vi "Frame Description FGV [Body Index].vi"(8 "error in (no error)":errorcluster, 9 "Command":enum16{"Get", "Set"}(ring)=enum."Set", 10 "FrameDescription":T1) -> (0 "error out":errorcluster, 2 "FrameDescription":T1)   [LabVIEW 2011, in "KinectOne.lvlib"]
uses:
  KinectOne.lvlib
  Type Defs/FrameDescription.ctl
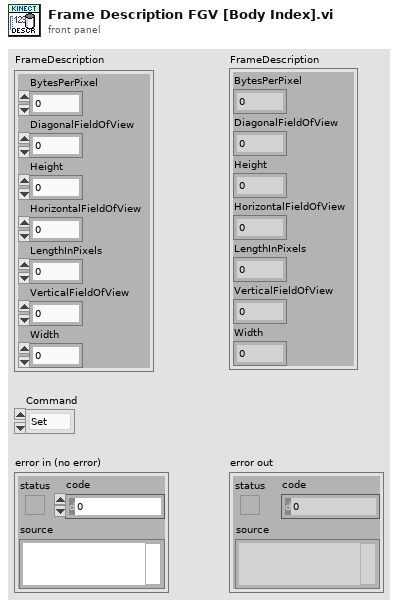
[diagram p1: front panel]
types:
  T1 = typedef "KinectOne.lvlib/FrameDescription.ctl" = cluster{"BytesPerPixel":u32, "DiagonalFieldOfView":sgl, "Height":i32, "HorizontalFieldOfView":sgl, "LengthInPixels":u32, "VerticalFieldOfView":sgl, "Width":i32}
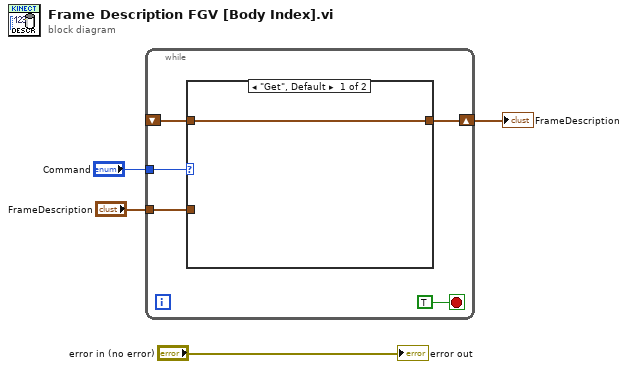
[diagram p0: block diagram]
diagram:
  n1 = while {
    tunnel: "Command" -> [w9]
    tunnel: "FrameDescription" -> [w7]
    shift-right: [w6] -> w1
    shift-left: _ -> [w5]
    stop <- TRUE stop-if-true
    n2 = case shown="\"Get\", Default" w9 {
      tunnel: w7 -> [_ w11]
      tunnel: [w10 w11] -> w6
      tunnel: w5 -> [w10 _]
      frame "Get", Default {
      }
      frame "Set" {
      }
    }
  }
  "FrameDescription" <- w1
  "error out" <- "error in (no error)"
